vi "DataLog.vi"() -> ()   [LabVIEW 2021]
panel:
  in  "Stop Button":bool
  out "AverageData":dbl
  out "RawData":dbl
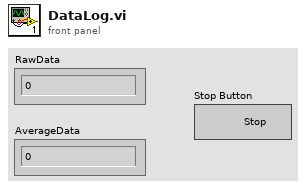
[diagram p1: front panel]
types:
  T1 = enum16{"open", "replace", "create", "open or create", "replace or create", "replace or create with confirmation"}
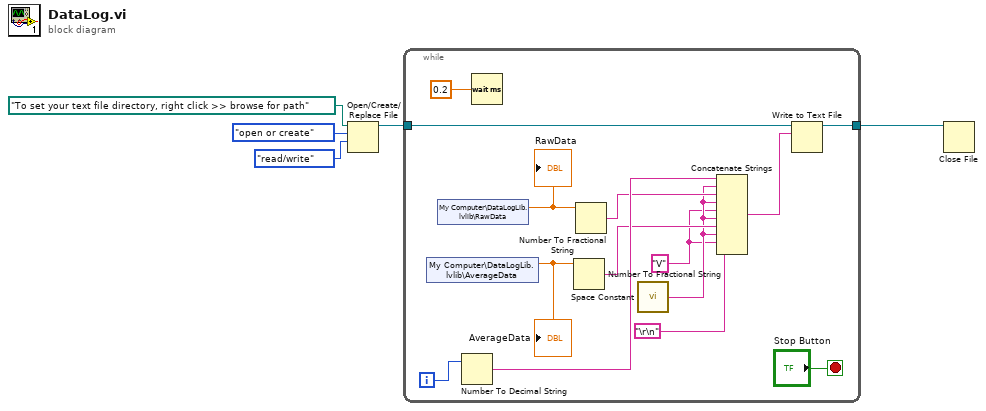
[diagram p0: block diagram]
diagram:
  n1 = Open/Create/Replace File(file path (use dialog)=path "To set your text file directory, right click >> browse for path", operation (0:open)=T1."open or create", access (0:read/write)=enum16{"read/write", "read-only", "write-only"}."read/write") -> (refnum out=w2:refnum<file>)  [unwired: 3 in, 2 out]
  n2 = while {
    tunnel: w2 -> [w19]
    tunnel: [w18] -> w1
    i -> [w17]
    stop <- "Stop Button" stop-if-true
    w11 = "V"
    n3 = shared-variable "My Computer\\DataLogLib.lvlib\\AverageData"() -> (w8:dbl)  [unwired: 1 in, 1 out]
    "AverageData" <- w8
    n4 = shared-variable "My Computer\\DataLogLib.lvlib\\RawData"() -> (w16:dbl)  [unwired: 1 in, 1 out]
    "RawData" <- w16
    n5 = Number To Decimal String(number=w17) -> (decimal integer string=w15:string)  [unwired: 1 in]
    n6 = Wait (ms)(milliseconds to wait=0.2) -> ()  [unwired: 1 out]
    n7 = Number To Fractional String(number=w8) -> (F-format string=w13:string)  [unwired: 3 in]
    n8 = Number To Fractional String(number=w16) -> (F-format string=w14:string)  [unwired: 3 in]
    n9 = call <vilib>:"Space Constant.vi"() -> ("String"=w12:string)
    n10 = Concatenate Strings(w15, w12, w14, w12, w11, w12, w13, w12, w11, "\r\n") -> (w9:string)
    n11 = Write to Text File(file (use dialog)=w19, text=w9) -> (refnum out=w18:refnum<file>)  [unwired: 2 in, 2 out]
  }
  n12 = Close File(refnum=w1) -> ()  [unwired: 1 in, 2 out]
